vi "GameInitTest.vi"() -> ()   [LabVIEW 2025]
panel:
  out "Field Display":picture
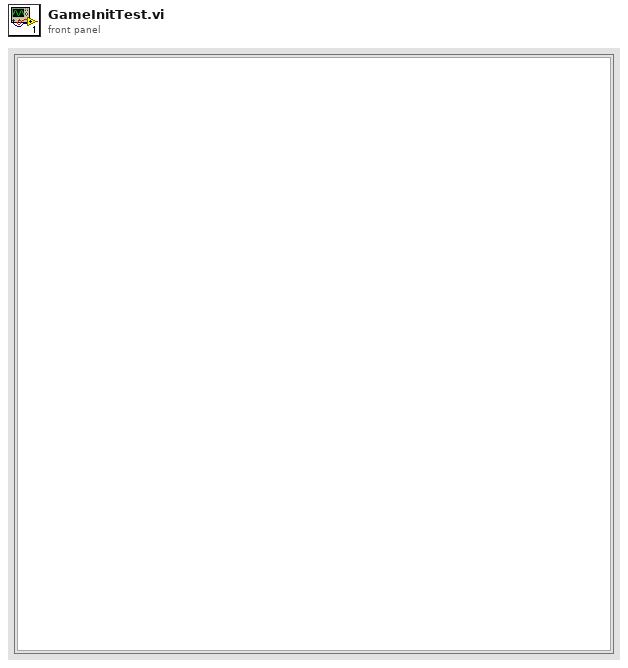
[diagram p1: front panel]
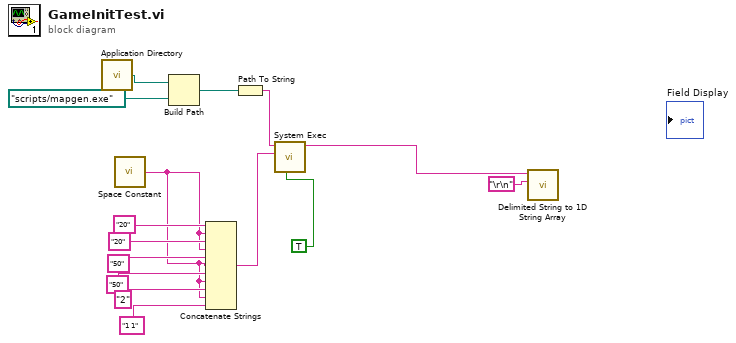
[diagram p0: block diagram]
diagram:
  n1 = call <vilib>:"Application Directory.vi"() -> ("Application Directory"=w13:path)
  n2 = call <vilib>:"Space Constant.vi"() -> ("String"=w4:string)
  n3 = Build Path(base path=w13, name or relative path=path "scripts/mapgen.exe") -> (appended path=w15:path)
  n4 = Concatenate Strings("20" ("string"), w4, "20" ("string"), w4, "50" ("string"), w4, "50" ("string"), w4, "2" ("string"), w4, "1 1" ("string")) -> (w11:string)
  n5 = Path To String(path=w15) -> (string=w12:string)
  n6 = call <vilib>:"System Exec.vi"("run minimized? (F)"=TRUE, "standard input"=w11, "command line"=w12) -> ("standard output"=w1:string)  [unwired: 5 in, 3 out]
  n7 = call <vilib>:"Delimited String to 1D String Array.vi"("delimiter"="\r\n", "delimited string"=w1) -> ()  [unwired: 9 in, 1 out]
